vi "Grayscale Frame Read.vi"(8 "error in (no error)":errorcluster, 11 "Video Frame in":refnum<class "Video Frame.lvclass">) -> (0 "error out":errorcluster, 2 "Image":T1, 3 "Video Frame out":refnum<class "Video Frame.lvclass">)   [LabVIEW 2018, in "Video Frame.lvclass"]
uses:
  Video Frame.lvclass
  <vilib>/vision/Image Controls.llb/IMAQ Image.ctl
  Video Frame.lvclass/Video Frame.ctl
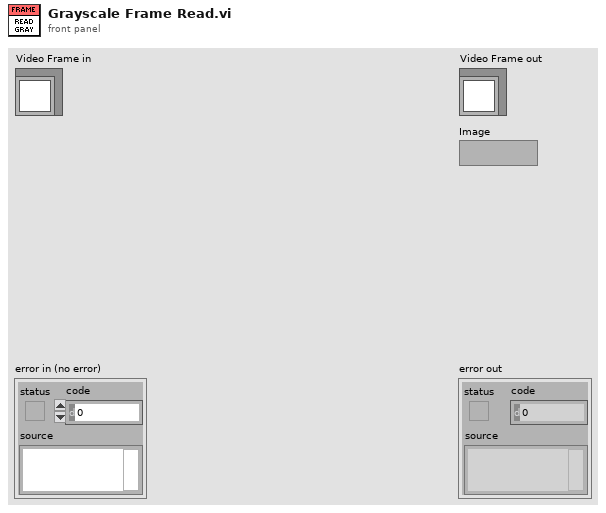
[diagram p1: front panel]
types:
  T1 = typedef "IMAQ Image.ctl" = refnum<image>
  T2 = typedef "Image Type" = u32
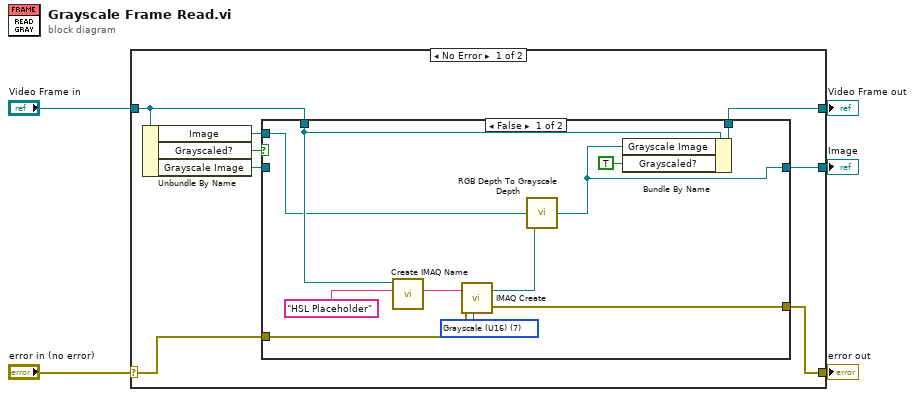
[diagram p0: block diagram]
diagram:
  n1 = case shown="No Error" "error in (no error)" {
    selector: "error in (no error)" -> [w8 w29]
    tunnel: [w9 w29] -> w4
    tunnel: [w6 w28] -> w2
    tunnel: "Video Frame in" -> [w7 w28]
    tunnel: [w11 _] -> w1
    frame No Error {
      n2 = Unbundle By Name(w7) -> ("Image"=w10:T1, "Grayscaled?"=w13:bool, "Grayscale Image"=w12:T1)
      n3 = case shown="False" w13 {
        tunnel: w12 -> [_ w27]
        tunnel: [w15 w27] -> w11
        tunnel: w10 -> [w17 _]
        tunnel: [w14 w26] -> w9
        tunnel: w8 -> [w23 w26]
        tunnel: w7 -> [w20 w25]
        tunnel: [w21 w25] -> w6
        frame False {
          w24 = T2 7 items=["Grayscale (U8)", "Grayscale (I16)", "Grayscale (SGL)", "Complex (CSG)", "RGB (U32)", "HSL (U32)", "RGB (U64)", "Grayscale (U16)"] ("Image Type")
          n4 = call-dynamic "Create IMAQ Name.vi"("Name (\"\")"="HSL Placeholder" ("input 2"), "Video Frame in"=w20) -> ("Name Out"=w18:string)  [unwired: 7 in, 2 out]
          n5 = call "IMAQ Create"("Image Name"=w18, "Image Type"=w24, "error in (no error)"=w23) -> ("New Image"=w16:T1, "error out"=w14:errorcluster)  [unwired: 2 in]
          n6 = call "RGB Depth To Grayscale Depth.vi"("Image Dest."=w16, "RGB Depth Image"=w17) -> ("Grayscale Depth Image"=w15:T1)  [unwired: 1 in]
          n7 = Bundle By Name(cluster=w20, "Grayscale Image"=w15, "Grayscaled?"=TRUE) -> (w21:refnum<class "Video Frame.lvclass">)
        }
        frame True {
        }
      }
    }
    frame Error {
    }
  }
  "error out" <- w4
  "Video Frame out" <- w2
  "Image" <- w1
